vi "Data.OnCompile.Execute.vi"(8 "error in":errorcluster, 10 "VS Ref Groups":T2(array[cluster]) {"VS Refs" format="%.0x"}, 11 "Custom Device Ref":T1 format="%.0x") -> (0 "error out":errorcluster, 3 "Custom Device Ref":T1 format="%.0x")   [LabVIEW 2015, in "Data Access System Explorer.lvlib"]
uses:
  Data Access System Explorer.lvlib
  <vilib>/NI Veristand/Custom Device API/Custom Device Item Ref.ctl
  <vilib>/NI Veristand/Custom Device API/Block Data Reference.ctl
  <vilib>/NI Veristand/Custom Device API/Data Reference.ctl
  <vilib>/NI Veristand/Custom Device API/Data Access Type.ctl
  <vilib>/NI Veristand/Custom Device API/Set Item Property (Variant).vi
  <vilib>/NI Veristand/Custom Device API/Custom Device API.lvlib
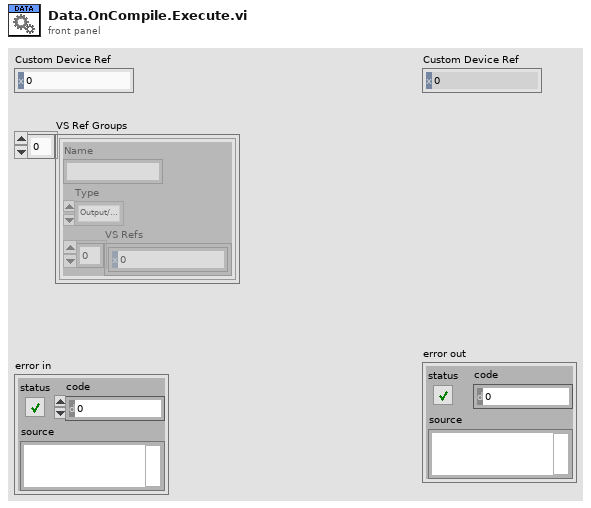
[diagram p1: front panel]
types:
  T1 = typedef "Custom Device API.lvlib/Custom Device Item Ref.ctl" = u64
  T2 = cluster{"Name":string, "Type":enum16{"Output/Write", "Input/Read", "Input/ReadWrite"}, "VS Refs":T1[]}[]
  T3 = typedef "Custom Device API.lvlib/Data Reference.ctl" = i32
  T4 = typedef "Custom Device API.lvlib/Block Data Reference.ctl" = cluster{"Data Reference":T3, "Offset":u64, "Length":u64}
  T5 = cluster{"Refs":T3[], "Values":dbl[], "Reset Values":dbl[]}[]
  T6 = cluster{"Read":cluster{"Refs":T4[], "Values":dbl[]}[], "Write":cluster{"Refs":T3[], "Values":dbl[]}[], "ReadWrite":cluster{"Refs":T3[], "Values":dbl[], "Reset Values":dbl[]}[], "LUT":variant}
  T7 = typedef "Custom Device API.lvlib/Data Access Type.ctl" = enum16{"Read", "Write"}
  T8 = cluster{"Refs":T3[], "Values":dbl[], "Reset Values":dbl[]}
  T9 = enum16{"Output/Write", "Input/Read", "Input/ReadWrite"}
  T10 = typedef "Custom Device API.lvlib/Custom Device Channel.ctl" = cluster{"Type":T11, "Units":string, "Default Value":dbl, "Faultable":bool, "Scalable":bool}
  T11 = typedef "Custom Device API.lvlib/Custom Device Channel Type.ctl" = enum16{"Input", "Output"}
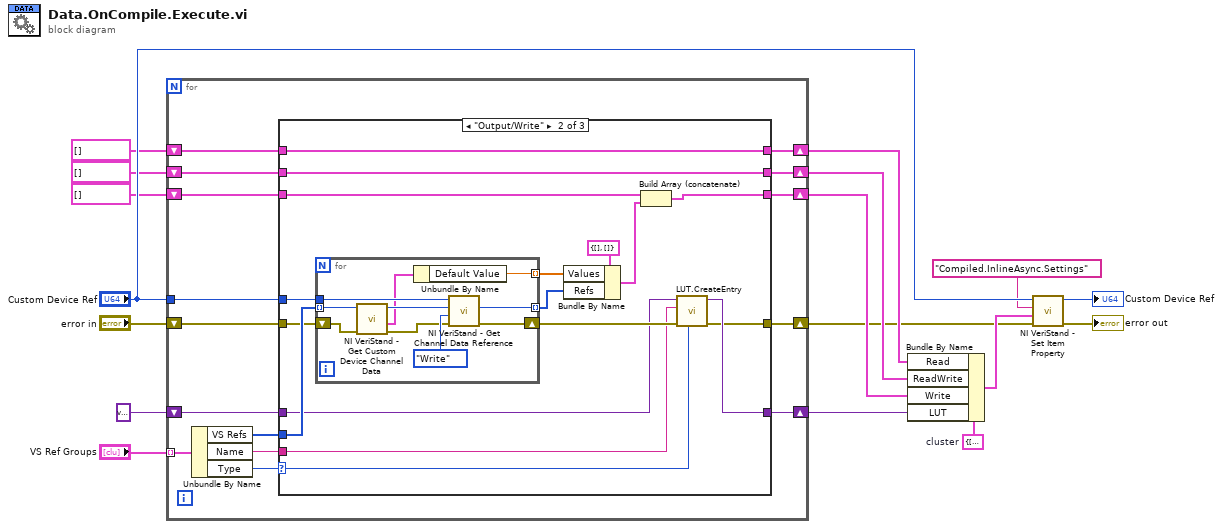
[diagram p0: block diagram]
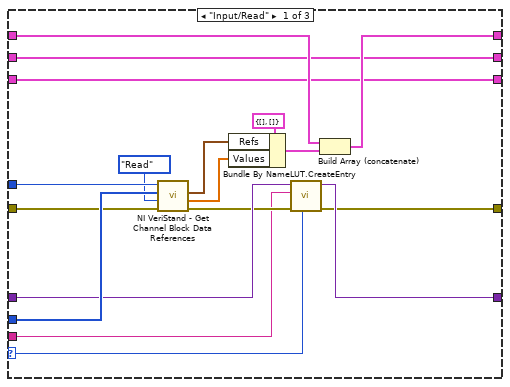
[diagram p2: hidden frame]
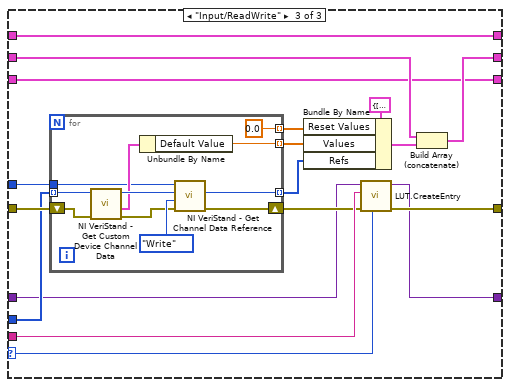
[diagram p3: hidden frame]
diagram:
  w13 = T6 {"Read"=[], "Write"=[], "ReadWrite"=[], "LUT"=variant}  # cluster
  n1 = for {
    tunnel: "VS Ref Groups" -> [w32] mode=indexing
    shift-right: [w30] -> w1
    shift-left: "error in" -> [w31]
    tunnel: "Custom Device Ref" -> [w28]
    shift-right: [w26] -> w2
    shift-left: variant ("LUT") -> [w27]
    shift-right: [w25] -> w4
    shift-left: cluster{"Refs":T4[], "Values":dbl[]}[] [] -> [w20]
    shift-right: [w22] -> w3
    shift-left: T5 [] -> [w21]
    shift-right: [w19] -> w5
    shift-left: cluster{"Refs":T3[], "Values":dbl[]}[] [] -> [w18]
    n2 = Unbundle By Name(w32) -> ("VS Refs"=w29:T1[], "Name"=w24:string, "Type"=w23:T9)
    n3 = case shown="\"Output/Write\"" w23 {
      selector: w23 -> [w38 w56 w88]
      tunnel: w31 -> [w47 w62 w92]
      tunnel: [w45 w57 w86] -> w30
      tunnel: w29 -> [w50 w67 w90]
      tunnel: w28 -> [w49 w66 w83]
      tunnel: w27 -> [w48 w59 w85]
      tunnel: [w46 w58 w84] -> w26
      tunnel: [w35 w54 w78] -> w25
      tunnel: w24 -> [w39 w60 w89]
      tunnel: [w34 w55 w80] -> w22
      tunnel: w21 -> [w34 w55 w82]
      tunnel: w20 -> [w37 w54 w78]
      tunnel: [w33 w52 w79] -> w19
      tunnel: w18 -> [w33 w51 w79]
      frame "Input/Read" {
        n4 = call <vilib>:"NI VeriStand - Get Channel Block Data References.vi"("error in (no error)"=w47, "Access"=Data_Access_Type."Read", "Channel Refs"=w50, "Device Ref in"=w49) -> ("error out"=w41:errorcluster, "Values Array"=w42:dbl[], "Block Data Refs"=w43:T4[])  [unwired: 4 in, 1 out]
        n5 = Bundle By Name(cluster=cluster{"Refs":T4[], "Values":dbl[]} {"Refs"=[], "Values"=[]}, "Refs"=w43, "Values"=w42) -> (w36:cluster{"Refs":T4[], "Values":dbl[]})
        n6 = call "LUT.CreateEntry.vi"("Type"=w38, "error in (no error)"=w41, "Name"=w39, "LUT"=w48) -> ("error out"=w45:errorcluster, "LUT"=w46:variant)  [unwired: 6 in]
        n7 = Build Array (concatenate)(w37, w36) -> (w35:cluster{"Refs":T4[], "Values":dbl[]}[])
      }
      frame "Output/Write" {
        n8 = for {
          tunnel: w66 -> [w76]
          tunnel: w67 -> [w75] mode=indexing
          shift-right: [w68] -> w61
          shift-left: w62 -> [w73]
          tunnel: [w71] -> w63 mode=indexing
          tunnel: [w70] -> w64 mode=indexing
          n9 = call <vilib>:"NI VeriStand - Get Custom Device Channel Data.vi"("error in (no error)"=w73, "Channel Ref in"=w75) -> ("error out"=w69:errorcluster, "Channel"=w72:T10, "Channel Ref out"=w74:T1)  [unwired: 4 in, 3 out]
          n10 = Unbundle By Name(w72) -> ("Default Value"=w71:dbl)
          n11 = call <vilib>:"NI VeriStand - Get Channel Data Reference.vi"("error in (no error)"=w69, "Access"=Data_Access_Type."Write", "Channel Ref in"=w74, "Device Ref in"=w76) -> ("error out"=w68:errorcluster, "Channel Data Reference"=w70:T3)  [unwired: 5 in, 1 out]
        }
        n12 = Bundle By Name(cluster=cluster{"Refs":T3[], "Values":dbl[]} {"Refs"=[], "Values"=[]}, "Values"=w63, "Refs"=w64) -> (w53:cluster{"Refs":T3[], "Values":dbl[]})
        n13 = Build Array (concatenate)(w51, w53) -> (w52:cluster{"Refs":T3[], "Values":dbl[]}[])
        n14 = call "LUT.CreateEntry.vi"("Type"=w56, "error in (no error)"=w61, "Name"=w60, "LUT"=w59) -> ("error out"=w57:errorcluster, "LUT"=w58:variant)  [unwired: 6 in]
      }
      frame "Input/ReadWrite" {
        n15 = for {
          shift-right: [w105] -> w87
          shift-left: w92 -> [w103]
          tunnel: [w100] -> w95 mode=indexing
          tunnel: [w99] -> w94 mode=indexing
          tunnel: [0.0] -> w93 mode=indexing
          tunnel: w90 -> [w97] mode=indexing
          tunnel: w83 -> [w96]
          n16 = call <vilib>:"NI VeriStand - Get Custom Device Channel Data.vi"("error in (no error)"=w103, "Channel Ref in"=w97) -> ("error out"=w102:errorcluster, "Channel"=w101:T10, "Channel Ref out"=w104:T1)  [unwired: 4 in, 3 out]
          n17 = Unbundle By Name(w101) -> ("Default Value"=w100:dbl)
          n18 = call <vilib>:"NI VeriStand - Get Channel Data Reference.vi"("error in (no error)"=w102, "Access"=Data_Access_Type."Write", "Channel Ref in"=w104, "Device Ref in"=w96) -> ("error out"=w105:errorcluster, "Channel Data Reference"=w99:T3)  [unwired: 5 in, 1 out]
        }
        n19 = Bundle By Name(cluster=T8 {"Refs"=[], "Values"=[], "Reset Values"=[]}, "Reset Values"=w93, "Values"=w95, "Refs"=w94) -> (w81:T8)
        n20 = call "LUT.CreateEntry.vi"("Type"=w88, "error in (no error)"=w87, "Name"=w89, "LUT"=w85) -> ("error out"=w86:errorcluster, "LUT"=w84:variant)  [unwired: 6 in]
        n21 = Build Array (concatenate)(w82, w81) -> (w80:T5)
      }
    }
  }
  n22 = Bundle By Name(cluster=w13, "Read"=w4, "ReadWrite"=w3, "Write"=w5, "LUT"=w2) -> (w14:T6)
  n23 = call-poly <vilib>:"NI VeriStand - Set Item Property.vi"("error in (no error)"=w1, "Value"=w14, "Property Name"="Compiled.InlineAsync.Settings", "Item Ref in"="Custom Device Ref") -> ("error out"=→"error out":errorcluster, "Item Ref out"=→"Custom Device Ref":T1)  [unwired: 5 in, 1 out]
